vi "multi assert test.vi"() -> ()   [LabVIEW 2016]
uses:
  <vilib>/Utility/traverseref.llb/TRef TravTarget.ctl
  <vilib>/Utility/traverseref.llb/VI Scripting - Traverse.lvlib
panel:
  out "size(s)":i32
  out "Numeric 4":dbl
  out "Numeric 3":i32
  out "String 2":string
  out "Boolean 2":bool
  in  "Boolean":bool
  in  "String":string
  in  "Numeric 2":i32
  in  "Numeric":dbl
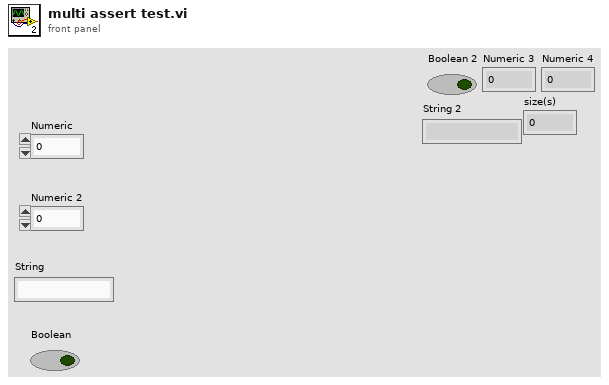
[diagram p1: front panel]
types:
  T1 = typedef "TRef TravTarget.ctl" = enum16{"FP", "BD", "Other"}
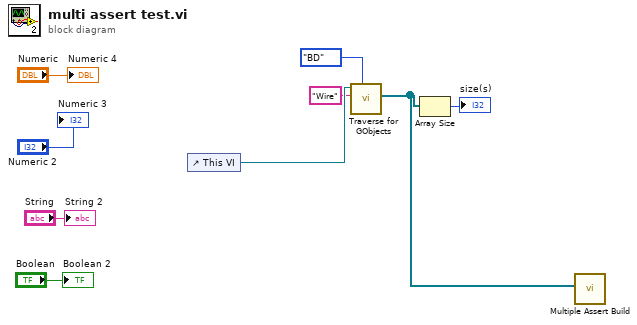
[diagram p0: block diagram]
diagram:
  n1 = control-ref of="This VI"() -> (w5:refnum<vi>)
  n2 = call <vilib>:"Traverse for GObjects.vi"("Traverse Target"=TRef_TravTarget."BD", "Class Name"="Wire", "VI Refnum"=w5) -> ("References"=w1:refnum<vi>[])  [unwired: 5 in, 3 out]
  n3 = Array Size(array=w1) -> (size(s)=→"size(s)":i32)
  n4 = call "Multiple Assert Build.vi"("GObj Array"=w1) -> ()  [unwired: 10 in, 1 out]
  "Boolean 2" <- "Boolean"
  "String 2" <- "String"
  "Numeric 3" <- "Numeric 2"
  "Numeric 4" <- "Numeric"
